vi "HFRR ADV v05 new software.vi"() -> ()   [LabVIEW 2025] (continued)
        n806 = local read "LIVE FEED MIN TEMP"() -> (w1181:bool)
        n807 = local write "LIVE FEED MAX TEMP"(TRUE ("LIVE FEED MAX TEMP")) -> ()
        n808 = local read "CAMERA ROI MIN TEMP"() -> (w1179:bool)
        n809 = case shown="True" w1181 {
          selector: w1181 -> [_ w1188]
          frame False {
          }
          frame True {
            n810 = Not(x=w1188) -> (.not. x?=w1187:bool)
            n811 = local write "LIVE FEED MIN TEMP"(w1187) -> ()
            n812 = call "CAMERA LIVE FEED FGV.vi"("Enum - Menu"=CAMERA_LIVE_FEED_ENUM."CAMERA MINIMIZE") -> ()  [unwired: 9 in, 2 out]
          }
        }
        n813 = case shown="True" w1179 {
          selector: w1179 -> [_ w1185]
          frame False {
          }
          frame True {
            n814 = Not(x=w1185) -> (.not. x?=w1184:bool)
            n815 = local write "CAMERA ROI MIN TEMP"(w1184) -> ()
            n816 = call "IMAGE ANALYSIS.vi"("Enum"=POST_ANALYSIS_ENUM."MINIMIZE UI") -> ()  [unwired: 9 in, 2 out]
          }
        }
        n817 = local write "CAMERA ROI MAX TEMP"(TRUE ("CAMERA ROI MAX TEMP")) -> ()
      }
      frame "About" {
        n818 = local read "LIVE FEED MIN TEMP"() -> (w1191:bool)
        n819 = local write "LIVE FEED MAX TEMP"(TRUE ("LIVE FEED MAX TEMP")) -> ()
        n820 = local read "CAMERA ROI MIN TEMP"() -> (w1190:bool)
        n821 = case shown="True" w1191 {
          selector: w1191 -> [_ w1198]
          frame False {
          }
          frame True {
            n822 = Not(x=w1198) -> (.not. x?=w1197:bool)
            n823 = local write "LIVE FEED MIN TEMP"(w1197) -> ()
            n824 = call "CAMERA LIVE FEED FGV.vi"("Enum - Menu"=CAMERA_LIVE_FEED_ENUM."CAMERA MINIMIZE") -> ()  [unwired: 9 in, 2 out]
          }
        }
        n825 = case shown="True" w1190 {
          selector: w1190 -> [_ w1195]
          frame False {
          }
          frame True {
            n826 = Not(x=w1195) -> (.not. x?=w1194:bool)
            n827 = local write "CAMERA ROI MIN TEMP"(w1194) -> ()
            n828 = call "IMAGE ANALYSIS.vi"("Enum"=POST_ANALYSIS_ENUM."MINIMIZE UI") -> ()  [unwired: 9 in, 2 out]
          }
        }
        n829 = local write "CAMERA ROI MAX TEMP"(TRUE ("CAMERA ROI MIN TEMP")) -> ()
      }
      frame "Advance" {
        n830 = local read "LIVE FEED MIN TEMP"() -> (w1201:bool)
        n831 = local write "LIVE FEED MAX TEMP"(TRUE ("LIVE FEED MAX TEMP")) -> ()
        n832 = local read "CAMERA ROI MIN TEMP"() -> (w1199:bool)
        n833 = case shown="True" w1201 {
          selector: w1201 -> [_ w1208]
          frame False {
          }
          frame True {
            n834 = Not(x=w1208) -> (.not. x?=w1207:bool)
            n835 = local write "LIVE FEED MIN TEMP"(w1207) -> ()
            n836 = call "CAMERA LIVE FEED FGV.vi"("Enum - Menu"=CAMERA_LIVE_FEED_ENUM."CAMERA MINIMIZE") -> ()  [unwired: 9 in, 2 out]
          }
        }
        n837 = local write "CAMERA ROI MAX TEMP"(TRUE ("CAMERA ROI MAX TEMP")) -> ()
        n838 = case shown="True" w1199 {
          selector: w1199 -> [_ w1205]
          frame False {
          }
          frame True {
            n839 = Not(x=w1205) -> (.not. x?=w1204:bool)
            n840 = local write "CAMERA ROI MIN TEMP"(w1204) -> ()
            n841 = call "IMAGE ANALYSIS.vi"("Enum"=POST_ANALYSIS_ENUM."MINIMIZE UI") -> ()  [unwired: 9 in, 2 out]
          }
        }
      }
      frame "Mooha" {
        n842 = local read "LIVE FEED MIN TEMP"() -> (w1211:bool)
        n843 = local write "LIVE FEED MAX TEMP"(TRUE ("LIVE FEED MAX TEMP")) -> ()
        n844 = local read "CAMERA ROI MIN TEMP"() -> (w1209:bool)
        n845 = case shown="True" w1211 {
          selector: w1211 -> [_ w1218]
          frame False {
          }
          frame True {
            n846 = Not(x=w1218) -> (.not. x?=w1217:bool)
            n847 = local write "LIVE FEED MIN TEMP"(w1217) -> ()
            n848 = call "CAMERA LIVE FEED FGV.vi"("Enum - Menu"=CAMERA_LIVE_FEED_ENUM."CAMERA MINIMIZE") -> ()  [unwired: 9 in, 2 out]
          }
        }
        n849 = local write "CAMERA ROI MAX TEMP"(TRUE ("CAMERA ROI MAX TEMP")) -> ()
        n850 = case shown="True" w1209 {
          selector: w1209 -> [_ w1215]
          frame False {
          }
          frame True {
            n851 = Not(x=w1215) -> (.not. x?=w1214:bool)
            n852 = local write "CAMERA ROI MIN TEMP"(w1214) -> ()
            n853 = call "IMAGE ANALYSIS.vi"("Enum"=POST_ANALYSIS_ENUM."MINIMIZE UI") -> ()  [unwired: 9 in, 2 out]
          }
        }
      }
    }
    n854 = local read "Auto Start Test"() -> (w960:bool)
    n855 = case shown="True" "sign in temp" {
      frame False {
      }
      frame True {
        w997 = 1 ("y")
        n856 = local read "USERNAME"() -> (w1003:string)
        n857 = local read "USER ID"() -> (w1000:string)
        n858 = call <vilib>:"Trim Whitespace.vi"("string"=w1003) -> ("trimmed string"=w1002:string)  [unwired: 1 in]
        n859 = call <vilib>:"Trim Whitespace.vi"("string"=w1000) -> ("trimmed string"=w1001:string)  [unwired: 1 in]
        n860 = String Length(string=w1002) -> (length=w999:i32)
        n861 = String Length(string=w1001) -> (length=w998:i32)
        n862 = Greater?(x=w999, y=w997) -> (0:w996:bool)
        n863 = Greater?(x=w998, y=w997) -> (0:w995:bool)
        n864 = And(x=w996, y=w995) -> (x .and. y?=w994:bool)
        n865 = case shown="True" w994 {
          frame False {
            n866 = property on="Sign In" class="Bool (strict)"("DisabledEnum"=T13."Disabled" ("Disabled")) -> ()  [unwired: 2 in, 2 out]
          }
          frame True {
            n867 = property on="Sign In" class="Bool (strict)"("DisabledEnum"=T13."Enabled" ("Disabled")) -> ()  [unwired: 2 in, 2 out]
          }
        }
      }
    }
    n868 = local read "Air Temperature"() -> (w977:bool)
    n869 = local read "Coefficient Of Friction"() -> (w978:bool)
    n870 = case shown="False" w960 {
      frame False {
        n871 = local read "Auto stop temp"() -> (w991:bool)
        n872 = case shown="True" w991 {
          frame False {
          }
          frame True {
            n873 = local write "Auto Start Temp"(FALSE ("Auto Start Temp")) -> ()
          }
        }
      }
      frame True {
        "Auto stop temp" <- TRUE ("Auto stop temp")
      }
    }
    n874 = local read "Humidity"() -> (w976:bool)
    n875 = case shown="\"HOME\"" w988 {
      frame "HOME" {
        n876 = local write "main tab sub"(enum32{"Page 1", "Page 2"}."Page 1" ("main tab sub")) -> ()
      }
      frame Default {
        n877 = local write "main tab sub"(enum32{"Page 1", "Page 2"}."Page 2" ("main tab sub")) -> ()
      }
    }
    n878 = case shown="True" w987 {
      selector: w987 -> [_ w1323]
      frame False {
      }
      frame True {
        n879 = Not(x=w1323) -> (.not. x?=w1322:bool)
        n880 = local write "Sign In"(w1322) -> ()
        n881 = local write "Main Dashboard Buttons"(T1."Test Setup" ("Main Dashboard Buttons")) -> ()
      }
    }
    n882 = case shown="\"Numeric Display\", Default" "Num/Graph" {
      frame "Numeric Display", Default {
        n883 = property on="Single/Multiple" class="RadioBtnsControl (strict)"("Visible"=FALSE) -> ()  [unwired: 2 in, 2 out]
        n884 = property on="Single - Graph" class="Ring (strict)"("Visible"=FALSE) -> ()  [unwired: 2 in, 2 out]
        n885 = local write "Main Tab Display"(T4."Dashboard 1" ("Main Tab Display")) -> ()
      }
      frame "Graph Display" {
        n886 = property on="Single/Multiple" class="RadioBtnsControl (strict)"("Visible"=TRUE) -> ()  [unwired: 2 in, 2 out]
        n887 = case shown="\"Multiple\"" "Single/Multiple" {
          frame "Single ", Default {
            n888 = property on="Single - Graph" class="Ring (strict)"("Visible"=TRUE) -> ()  [unwired: 2 in, 2 out]
            n889 = local write "Main Tab Display"(T4."Dashboard 3" ("Main Tab Display")) -> ()
          }
          frame "Multiple" {
            n890 = property on="Single - Graph" class="Ring (strict)"("Visible"=FALSE) -> ()  [unwired: 2 in, 2 out]
            n891 = local write "Main Tab Display"(T4."Dashboard 2" ("Main Tab Display")) -> ()
          }
        }
      }
    }
    n892 = local read "Stroke"() -> (w975:bool)
    n893 = local read "USERNAME"() -> (w981:string)
    n894 = local read "USER ID"() -> (w980:string)
    n895 = case shown="True" w978 {
      selector: w978 -> [_ w1258]
      frame False {
      }
      frame True {
        n896 = Not(x=w1258) -> (.not. x?=w1257:bool)
        n897 = local write "Coefficient Of Friction"(w1257) -> ()
        n898 = local write "Tab Control 2"(T6."Coefficient Of Friction" ("Tab Control 2")) -> ()
      }
    }
    n899 = case shown="True" w977 {
      selector: w977 -> [_ w1255]
      frame False {
      }
      frame True {
        n900 = Not(x=w1255) -> (.not. x?=w1253:bool)
        n901 = local write "Air Temperature"(w1253) -> ()
        n902 = local write "Tab Control 2"(T6."Air Temperature" ("Tab Control 2")) -> ()
      }
    }
    n903 = local write "Operator ID"(w980) -> ()
    n904 = case shown="True" w975 {
      selector: w975 -> [_ w1249]
      frame False {
      }
      frame True {
        n905 = Not(x=w1249) -> (.not. x?=w1247:bool)
        n906 = local write "Stroke"(w1247) -> ()
        n907 = local write "Tab Control 2"(T6."Stroke" ("Tab Control 2")) -> ()
      }
    }
    n908 = local write "tested by"(w981) -> ()
    n909 = case shown="True" w976 {
      selector: w976 -> [_ w1252]
      frame False {
      }
      frame True {
        n910 = Not(x=w1252) -> (.not. x?=w1250:bool)
        n911 = local write "Humidity"(w1250) -> ()
        n912 = local write "Tab Control 2"(T6."Humidity" ("Tab Control 2")) -> ()
      }
    }
    n913 = case shown="\"Advance\"" "Main Dashboard Buttons" {
      tunnel: [T2."HOME" ("Main Tab") T2."Test Setup" ("Main Tab") T2."Acquire" ("Main Tab") T2."Adv Scar" ("Main Tab") T2."Adv Scar Report" ("Main Tab") T2."Compare Files" ("Main Tab") T2."About" ("Main Tab") T2."Advance" ("Main Tab")] -> w985
      frame "Home", Default {
      }
      frame "Test Setup" {
      }
      frame "Dashboard" {
      }
      frame "Imaging" {
      }
      frame "Report" {
      }
      frame "Analysis" {
      }
      frame "About" {
      }
      frame "Advance" {
      }
    }
    n914 = Wait (ms)(milliseconds to wait=u32 100) -> ()  [unwired: 1 out]
    n915 = local read "Main Tab Display"() -> (w979:T4)
    n916 = local write "Main Tab"(w985) -> ()
    n917 = case shown="\"Dashboard 3\"" w979 {
      frame "Dashboard 1", Default {
        n918 = property on="Reset Graph" class="Bool (strict)"("Visible"=FALSE) -> ()  [unwired: 2 in, 2 out]
      }
      frame "Dashboard 2" {
        n919 = property on="Reset Graph" class="Bool (strict)"("Visible"=TRUE) -> ()  [unwired: 2 in, 2 out]
      }
      frame "Dashboard 3" {
        n920 = property on="Reset Graph" class="Bool (strict)"("Visible"=TRUE) -> ()  [unwired: 2 in, 2 out]
      }
    }
    n921 = local read "SCAR MEASURMENT"() -> (w967:enum32{"Auto Scar", "Manual Scar"})
    n922 = local read "Humidity"() -> (w982:bool)
    n923 = local read "Cap Live Image"() -> (w964:bool)
    n924 = local read "Sample Temperature"() -> (w974:bool)
    n925 = local read "Air Temp vs Humidity"() -> (w972:bool)
    n926 = local read "Frequency"() -> (w973:bool)
    n927 = case shown="False" w982 {
      frame False {
        n928 = local write "Humidity On Command"(TRUE ("Humidity On Command")) -> ()
        n929 = case shown="True" "Humidity Off Command" {
          selector: "Humidity Off Command" -> [_ w1265]
          frame False {
          }
          frame True {
            n930 = stacked-sequence {
              frame #0 {
                n931 = local read "WriteHumidity"() -> (w1267:string[])
                n932 = Insert Into Array(array=w1267, new element="R;1" ("new element/subarray")) -> (w1268:string[])  [unwired: 1 in]
                n933 = local write "WriteHumidity"(w1268) -> ()
              }
              frame #1 {
                n934 = Wait (ms)(milliseconds to wait=u32 2000) -> ()  [unwired: 1 out]
              }
              frame #2 {
                n935 = local read "EVENT LOG"() -> (w1274:string)
                n936 = local read "WriteHumidity"() -> (w1271:string[])
                n937 = call "Event Log.vi"("Content"="Humidity Control Off" ("string"), "EVENT LOG"=w1274) -> ("EVENT LOG"=w1275:string)  [unwired: 8 in, 1 out]
                n938 = local write "EVENT LOG"(w1275) -> ()
                n939 = Insert Into Array(array=w1271, new element="R;1" ("new element/subarray")) -> (w1272:string[])  [unwired: 1 in]
                n940 = local write "WriteHumidity"(w1272) -> ()
              }
            }
            n941 = Not(x=w1265) -> (.not. x?=w1264:bool)
            n942 = local write "Humidity Off Command"(w1264) -> ()
          }
        }
      }
      frame True {
        n943 = local write "Humidity Off Command"(TRUE ("Humidity Off Command")) -> ()
        n944 = case shown="False" "Humidity On Command" {
          selector: "Humidity On Command" -> [_ w1279]
          frame False {
          }
          frame True {
            n945 = stacked-sequence {
              frame #0 {
                n946 = local read "Set Rh"() -> (w1285:dbl)
                n947 = Number To Fractional String(number=w1285, precision (6)=i16 2) -> (F-format string=w1286:string)  [unwired: 2 in]
                n948 = local read "WriteHumidity"() -> (w1283:string[])
                n949 = Concatenate Strings("M;" ("new element/subarray"), w1286) -> (w1284:string)
                n950 = Insert Into Array(array=w1283, new element=w1284) -> (w1282:string[])  [unwired: 1 in]
                n951 = local write "WriteHumidity"(w1282) -> ()
              }
              frame #1 {
                n952 = Wait (ms)(milliseconds to wait=u32 1500) -> ()  [unwired: 1 out]
              }
              frame #2 {
                (unwired) "% RH" ("string")
                (unwired) i16 2 ("precision (6)")
                (unwired) "M;" ("new element/subarray")
                n953 = local read "Set Rh"() -> (w1293:dbl)
                n954 = Number To Fractional String(number=w1293, precision (6)=i16 2) -> (F-format string=w1290:string)  [unwired: 2 in]
                n955 = local read "WriteHumidity"() -> (w1295:string[])
                n956 = Concatenate Strings("M;" ("new element/subarray"), w1290) -> (w1294:string)
                n957 = Concatenate Strings("Humidity Set to : " ("string"), w1290, "% RH" ("string")) -> (w1288:string)
                n958 = Insert Into Array(array=w1295, new element=w1294) -> (w1296:string[])  [unwired: 1 in]
                n959 = disable-structure shown="Enabled" {
                  frame Enabled {
                    n960 = local read "EVENT LOG"() -> (w1299:string)
                    n961 = call "Event Log.vi"("Content"="Humidity Control On", "EVENT LOG"=w1299) -> ("EVENT LOG"=w1300:string)  [unwired: 8 in, 1 out]
                    n962 = local write "EVENT LOG"(w1300) -> ()
                  }
                  frame Disabled {
                  }
                }
                n963 = disable-structure shown="Enabled" {
                  disable-tunnel: w1288 -> [_ _]
                  frame Enabled {
                    n964 = local read "EVENT LOG"() -> (w1302:string)
                    n965 = call "Event Log.vi"("Content"="Humidity Control On", "EVENT LOG"=w1302) -> ("EVENT LOG"=w1303:string)  [unwired: 8 in, 1 out]
                    n966 = local write "EVENT LOG"(w1303) -> ()
                  }
                  frame Disabled {
                  }
                }
                n967 = local write "WriteHumidity"(w1296) -> ()
              }
            }
            n968 = Not(x=w1279) -> (.not. x?=w1278:bool)
            n969 = local write "Humidity On Command"(w1278) -> ()
          }
        }
      }
    }
    n970 = Equal?(x=w967, y=enum32{"Auto Scar", "Manual Scar"}."Auto Scar" ("SCAR MEASURMENT")) -> (x = y?=w963:bool)
    n971 = local read "TEST STANDARD"() -> (w970:T3)
    n972 = And(x=w964, y=w963) -> (x .and. y?=w965:bool)
    n973 = case shown="True" w965 {
      selector: w965 -> [_ w1064]
      tunnel: errorcluster {"status"=FALSE, "code"=0, "source"=""} ("error in (no error) 3") -> [_ w1065]
      frame False {
      }
      frame True {
        n974 = stacked-sequence {
          tunnel: w1065 -> [_ _ _ _ _ _ _ w1113]
          tunnel: w1064 -> [_ _ _ _ _ w1094 _ _]
          frame #0 {
            n975 = call "CAMERA LIVE FEED FGV.vi"("Enum - Menu"=CAMERA_LIVE_FEED_ENUM."CAMERA MINIMIZE") -> ()  [unwired: 9 in, 2 out]
          }
          frame #1 {
            n976 = property on="Auto Scar Check  2" class="Clust (strict)"("Visible"=TRUE) -> ()  [unwired: 2 in, 2 out]
          }
          frame #2 {
            n977 = String To Path(string="C:\\LAB-IQ\\Image Calibrate v01.dcf") -> (path=w1070:path)
            n978 = Open/Create/Replace File ("Open File")(file path (use dialog)=w1070) -> (refnum out=w1071:refnum<file>)  [unwired: 5 in, 2 out]
            n979 = for {
              N: 4 -> [_]
              tunnel: w1071 -> [w1077]
              i -> [w1073]
              n980 = Read from Text File ("Read File")(file (use dialog)=w1077) -> (text=w1078:string)  [unwired: 3 in, 3 out]
              n981 = String Subset(string=w1078, offset (0)=6, length (rest)=10 ("length (rest)")) -> (substring=w1074:string)
              n982 = Fract/Exp String To Number(string=w1074) -> (number=w1072:dbl)  [unwired: 3 in, 1 out]
              n983 = case shown="0" w1073 {
                tunnel: w1072 -> [w1079 w1080 _ w1081 _]
                frame 0 {
                  "5x Gain" <- w1079
                }
                frame 1 {
                  "10x Gain" <- w1080
                }
                frame 2 {
                }
                frame 3 {
                  "100x gain" <- w1081
                }
                frame 4, Default {
                }
              }
            }
          }
          frame #3 {
            n984 = local read "FILE 3"() -> (w1087:string)
            n985 = call <vilib>:"Trim Whitespace.vi"("string"="C:\\LAB-IQ\\images\\") -> ("trimmed string"=w1089:string)  [unwired: 1 in]
            n986 = String To Path(string=w1089) -> (path=w1088:path)
            n987 = Concatenate Strings(w1087, ".png" ("string")) -> (w1086:string)
            n988 = Build Path(base path=w1088, name or relative path=w1086) -> (appended path=w1084:path)
            "Image path" <- w1084
            n989 = Path To String(path=w1084) -> (string=w1083:string)
            n990 = call "CAMERA LIVE FEED FGV.vi"("Enum - Menu"=CAMERA_LIVE_FEED_ENUM."CAMERA SAVE", "Image Path"=w1083) -> ()  [unwired: 8 in, 2 out]
          }
          frame #4 {
            n991 = One Button Dialog(message="Image saved successfully") -> ()  [unwired: 1 in, 1 out]
          }
          frame #5 {
            n992 = local read "TEST STANDARD"() -> (w1093:T3)
            n993 = local read "Magnification len live scar"() -> (w1105:string)
            n994 = Not(x=w1094) -> (.not. x?=w1095:bool)
            n995 = local write "Cap Live Image"(w1095) -> ()
            n996 = case shown="\"ISO 12156\"" w1093 {
              tunnel: ["ASTM D6079" "ISO 12156"] -> w1092
              frame "ASTM D6079", Default {
              }
              frame "ISO 12156" {
              }
            }
            n997 = case shown="\"5x\", Default" w1105 {
              tunnel: [w1108 w1109] -> w1104
              frame "5x", Default {
                n998 = local read "5x Gain"() -> (w1108:dbl)
              }
              frame "10x" {
                # "5x"
                n999 = local read "10x Gain"() -> (w1109:dbl)
              }
            }
            n1000 = local read "Image path"() -> (w1103:path)
            n1001 = local read "FILE 3"() -> (w1096:string)
            n1002 = call "EDGE DETCTION.vi"("GAIN VALUE"=w1104, "Image Path"=w1103) -> ("error out"=w1102:errorcluster, "return value"=w1101:cluster{string, string, dbl, dbl, dbl})  [unwired: 8 in]
            n1003 = Bundle By Name(cluster=T18 {"File Name"="", "Test Method"="", "Operator"="", "Fuel Description"="", "Date and time"=""} ("Main Ref"), "File Name"=w1096, "Test Method"=w1092) -> (w1097:T18)
            n1004 = call "duf file read.vi"("error in (no error)"=w1102, "Main Ref"=w1097) -> ("error out"=w1100:errorcluster, "Main Ref 2"=w1098:T18)  [unwired: 8 in]
            n1005 = call "EDGE DETECTION REPORT.vi"("error in (no error)"=w1100, "return value 2"=w1101, "Main Ref"=w1098) -> ()  [unwired: 8 in, 1 out]
          }
          frame #6 {
            n1006 = property on="Auto Scar Check  2" class="Clust (strict)"("Visible"=FALSE) -> ()  [unwired: 2 in, 2 out]
          }
          frame #7 {
            n1007 = call "CAMERA LIVE FEED FGV.vi"("Enum - Menu"=CAMERA_LIVE_FEED_ENUM."CAMERA MINIMIZE", "error in (no error)"=w1113) -> ()  [unwired: 8 in, 2 out]
            n1008 = local write "Main Dashboard Buttons"(T1."Home" ("Main Dashboard Buttons")) -> ()
            n1009 = local write "Main Tab"(T2."HOME" ("Main Tab")) -> ()
          }
        }
      }
    }
    n1010 = local read "Heater Button"() -> (w971:bool)
    n1011 = case shown="True" w973 {
      selector: w973 -> [_ w1243]
      frame False {
      }
      frame True {
        n1012 = Not(x=w1243) -> (.not. x?=w1241:bool)
        n1013 = local write "Frequency"(w1241) -> ()
        n1014 = local write "Tab Control 2"(T6."Frequency" ("Tab Control 2")) -> ()
      }
    }
    n1015 = case shown="True" w972 {
      selector: w972 -> [_ w1240]
      frame False {
      }
      frame True {
        n1016 = Not(x=w1240) -> (.not. x?=w1238:bool)
        n1017 = local write "Air Temp vs Humidity"(w1238) -> ()
        n1018 = local write "Tab Control 2"(T6."Air Temp vs Rh" ("Tab Control 2")) -> ()
      }
    }
    n1019 = case shown="True" w974 {
      selector: w974 -> [_ w1246]
      frame False {
      }
      frame True {
        n1020 = Not(x=w1246) -> (.not. x?=w1244:bool)
        n1021 = local write "Sample Temperature"(w1244) -> ()
        n1022 = local write "Tab Control 2"(T6."Sample Temperature" ("Tab Control 2")) -> ()
      }
    }
    n1023 = case shown="\"Custom\"" w970 {
      frame "ASTM D6079", Default {
        w1219 = "ASTM D6079 TEST CONDITIONS" ("Standard 2")
        n1024 = local write "Standard 2"(w1219) -> ()
        n1025 = local write "Standard"(w1219) -> ()
      }
      frame "ISO 12156" {
        w1220 = "ISO 12156 TEST CONDITIONS" ("Standard 2")
        n1026 = local write "Standard 2"(w1220) -> ()
        n1027 = local write "Standard"(w1220) -> ()
      }
      frame "CEC F-096-A-06" {
        w1221 = "CEC F-096-A-06 TEST CONDITIONS" ("Standard 2")
        n1028 = local write "Standard 2"(w1221) -> ()
        n1029 = local write "Standard"(w1221) -> ()
      }
      frame "Custom" {
        w1222 = "CUSTOM TEST CONDITIONS" ("Standard 2")
        n1030 = local write "Standard 2"(w1222) -> ()
        n1031 = local write "Standard"(w1222) -> ()
      }
    }
    n1032 = case shown="True" w971 {
      frame False {
        n1033 = local write "Temperature On Command"(TRUE ("Temperature On Command")) -> ()
        n1034 = case shown="True" "Temperature Off Command" {
          selector: "Temperature Off Command" -> [_ w1226]
          frame False {
          }
          frame True {
            n1035 = Not(x=w1226) -> (.not. x?=w1225:bool)
            n1036 = local read "EVENT LOG"() -> (w1229:string)
            n1037 = local write "Temperature Off Command"(w1225) -> ()
            n1038 = call "Event Log.vi"("Content"="Heater Off", "EVENT LOG"=w1229) -> ("EVENT LOG"=w1228:string)  [unwired: 8 in, 1 out]
            n1039 = local write "EVENT LOG"(w1228) -> ()
          }
        }
      }
      frame True {
        n1040 = local write "Temperature Off Command"(TRUE ("Temperature Off Command")) -> ()
        n1041 = case shown="True" "Temperature On Command" {
          selector: "Temperature On Command" -> [_ w1233]
          frame False {
          }
          frame True {
            n1042 = Not(x=w1233) -> (.not. x?=w1232:bool)
            n1043 = local write "Temperature On Command"(w1232) -> ()
            n1044 = disable-structure shown="Enabled" {
              disable-tunnel: "Heater On" -> [w1235 _]
              frame Enabled {
                n1045 = local read "EVENT LOG"() -> (w1236:string)
                n1046 = call "Event Log.vi"("Content"=w1235, "EVENT LOG"=w1236) -> ("EVENT LOG"=w1237:string)  [unwired: 8 in, 1 out]
                n1047 = local write "EVENT LOG"(w1237) -> ()
              }
              frame Disabled {
              }
            }
          }
        }
      }
    }
    n1048 = local read "Main Tab"() -> (w962:T2)
    n1049 = case shown="\"About\"" w962 {
      frame "HOME", Default {
        w1008 = T13."Enabled" ("Disabled")
        n1050 = local read "Service Password enable"() -> (w1007:bool)
        n1051 = property on="Imaging" class="Bool (strict)"("DisabledEnum"=w1008) -> ()  [unwired: 2 in, 2 out]
        n1052 = property on="Dashboard" class="Bool (strict)"("DisabledEnum"=w1008) -> ()  [unwired: 2 in, 2 out]
        n1053 = property on="Test Setup" class="Bool (strict)"("DisabledEnum"=w1008) -> ()  [unwired: 2 in, 2 out]
        n1054 = property on="Analysis" class="Bool (strict)"("DisabledEnum"=w1008) -> ()  [unwired: 2 in, 2 out]
        n1055 = property on="Home" class="Bool (strict)"("DisabledEnum"=w1008) -> ()  [unwired: 2 in, 2 out]
        n1056 = property on="Report" class="Bool (strict)"("DisabledEnum"=w1008) -> ()  [unwired: 2 in, 2 out]
        n1057 = property on="Main Dashboard Buttons" class="RadioBtnsControl (strict)"("DisabledEnum"=w1008) -> ()  [unwired: 2 in, 2 out]
        n1058 = case shown="True" w1007 {
          tunnel: [T13."Disabled" ("Disabled") T13."Enabled" ("Disabled")] -> w1006
          frame False {
          }
          frame True {
          }
        }
        n1059 = property on="About" class="Bool (strict)"("DisabledEnum"=w1006) -> ()  [unwired: 2 in, 2 out]
      }
      frame "Test Setup" {
        w1013 = T13."Enabled" ("Disabled")
        n1060 = local read "Service Password enable"() -> (w1012:bool)
        n1061 = property on="Dashboard" class="Bool (strict)"("DisabledEnum"=T13."Disabled" ("Disabled")) -> ()  [unwired: 2 in, 2 out]
        n1062 = property on="Imaging" class="Bool (strict)"("DisabledEnum"=w1013) -> ()  [unwired: 2 in, 2 out]
        n1063 = property on="Analysis" class="Bool (strict)"("DisabledEnum"=w1013) -> ()  [unwired: 2 in, 2 out]
        n1064 = property on="Home" class="Bool (strict)"("DisabledEnum"=w1013) -> ()  [unwired: 2 in, 2 out]
        n1065 = property on="Report" class="Bool (strict)"("DisabledEnum"=w1013) -> ()  [unwired: 2 in, 2 out]
        n1066 = property on="Test Setup" class="Bool (strict)"("DisabledEnum"=w1013) -> ()  [unwired: 2 in, 2 out]
        n1067 = case shown="True" w1012 {
          tunnel: [T13."Disabled" ("Disabled") T13."Enabled" ("Disabled")] -> w1011
          frame False {
          }
          frame True {
          }
        }
        n1068 = property on="About" class="Bool (strict)"("DisabledEnum"=w1011) -> ()  [unwired: 2 in, 2 out]
      }
      frame "Adv Scar" {
        w1020 = T13."Enabled" ("Disabled")
        n1069 = property on="Dashboard" class="Bool (strict)"("DisabledEnum"=T13."Disabled" ("Disabled")) -> ()  [unwired: 2 in, 2 out]
        n1070 = property on="Imaging" class="Bool (strict)"("DisabledEnum"=w1020) -> ()  [unwired: 2 in, 2 out]
        n1071 = property on="Analysis" class="Bool (strict)"("DisabledEnum"=w1020) -> ()  [unwired: 2 in, 2 out]
        n1072 = property on="Home" class="Bool (strict)"("DisabledEnum"=w1020) -> ()  [unwired: 2 in, 2 out]
        n1073 = property on="Report" class="Bool (strict)"("DisabledEnum"=w1020) -> ()  [unwired: 2 in, 2 out]
        n1074 = property on="Test Setup" class="Bool (strict)"("DisabledEnum"=w1020) -> ()  [unwired: 2 in, 2 out]
        n1075 = local read "Service Password enable"() -> (w1018:bool)
        n1076 = case shown="True" w1018 {
          tunnel: [T13."Disabled" ("Disabled") T13."Enabled" ("Disabled")] -> w1017
          frame False {
          }
          frame True {
          }
        }
        n1077 = property on="About" class="Bool (strict)"("DisabledEnum"=w1017) -> ()  [unwired: 2 in, 2 out]
      }
      frame "Adv Scar Report" {
        w1025 = T13."Enabled" ("Disabled")
        n1078 = property on="Dashboard" class="Bool (strict)"("DisabledEnum"=T13."Disabled" ("Disabled")) -> ()  [unwired: 2 in, 2 out]
        n1079 = property on="Imaging" class="Bool (strict)"("DisabledEnum"=w1025) -> ()  [unwired: 2 in, 2 out]
        n1080 = property on="Analysis" class="Bool (strict)"("DisabledEnum"=w1025) -> ()  [unwired: 2 in, 2 out]
        n1081 = property on="Home" class="Bool (strict)"("DisabledEnum"=w1025) -> ()  [unwired: 2 in, 2 out]
        n1082 = property on="Report" class="Bool (strict)"("DisabledEnum"=w1025) -> ()  [unwired: 2 in, 2 out]
        n1083 = property on="Test Setup" class="Bool (strict)"("DisabledEnum"=w1025) -> ()  [unwired: 2 in, 2 out]
        n1084 = local read "Service Password enable"() -> (w1024:bool)
        n1085 = case shown="True" w1024 {
          tunnel: [T13."Disabled" ("Disabled") T13."Enabled" ("Disabled")] -> w1023
          frame False {
          }
          frame True {
          }
        }
        n1086 = property on="About" class="Bool (strict)"("DisabledEnum"=w1023) -> ()  [unwired: 2 in, 2 out]
      }
      frame "Compare Files" {
        w1031 = T13."Enabled" ("Disabled")
        n1087 = local read "Service Password enable"() -> (w1030:bool)
        n1088 = property on="Dashboard" class="Bool (strict)"("DisabledEnum"=T13."Disabled" ("Disabled")) -> ()  [unwired: 2 in, 2 out]
        n1089 = property on="Imaging" class="Bool (strict)"("DisabledEnum"=w1031) -> ()  [unwired: 2 in, 2 out]
        n1090 = property on="Analysis" class="Bool (strict)"("DisabledEnum"=w1031) -> ()  [unwired: 2 in, 2 out]
        n1091 = property on="Home" class="Bool (strict)"("DisabledEnum"=w1031) -> ()  [unwired: 2 in, 2 out]
        n1092 = property on="Report" class="Bool (strict)"("DisabledEnum"=w1031) -> ()  [unwired: 2 in, 2 out]
        n1093 = property on="Test Setup" class="Bool (strict)"("DisabledEnum"=w1031) -> ()  [unwired: 2 in, 2 out]
        n1094 = case shown="True" w1030 {
          tunnel: [T13."Disabled" ("Disabled") T13."Enabled" ("Disabled")] -> w1029
          frame False {
          }
          frame True {
          }
        }
        n1095 = property on="About" class="Bool (strict)"("DisabledEnum"=w1029) -> ()  [unwired: 2 in, 2 out]
      }
      frame "Acquire" {
        n1096 = local read "Service Password enable"() -> (w1035:bool)
        n1097 = property on="Test Setup" class="Bool (strict)"("DisabledEnum"=T13."Disabled" ("Disabled")) -> ()  [unwired: 2 in, 2 out]
        n1098 = local read "Auto Start Test"() -> (w1037:bool)
        n1099 = local read "RUN"() -> (w1039:bool)
        n1100 = case shown="True" w1035 {
          tunnel: [T13."Disabled" ("Disabled") T13."Enabled" ("Disabled")] -> w1036
          frame False {
          }
          frame True {
          }
        }
        n1101 = Or(x=w1039, y=w1037) -> (x .or. y?=w1038:bool)
        n1102 = case shown="True" w1038 {
          tunnel: [T13."Enabled" ("Disabled") T13."Disabled" ("Disabled")] -> w1041
          frame False {
          }
          frame True {
          }
        }
        n1103 = property on="About" class="Bool (strict)"("DisabledEnum"=w1036) -> ()  [unwired: 2 in, 2 out]
        n1104 = property on="Imaging" class="Bool (strict)"("DisabledEnum"=w1041) -> ()  [unwired: 2 in, 2 out]
        n1105 = property on="Dashboard" class="Bool (strict)"("DisabledEnum"=w1041) -> ()  [unwired: 2 in, 2 out]
        n1106 = property on="Analysis" class="Bool (strict)"("DisabledEnum"=w1041) -> ()  [unwired: 2 in, 2 out]
        n1107 = property on="Home" class="Bool (strict)"("DisabledEnum"=w1041) -> ()  [unwired: 2 in, 2 out]
        n1108 = property on="Report" class="Bool (strict)"("DisabledEnum"=w1041) -> ()  [unwired: 2 in, 2 out]
      }
      frame "About" {
        n1109 = local read "FILE"() -> (w1054:string)
        n1110 = local read "TEST FILE NAM,E SAVED"() -> (w1047:bool)
        n1111 = call <vilib>:"Trim Whitespace.vi"("string"=w1054) -> ("trimmed string"=w1053:string)  [unwired: 1 in]
        n1112 = local read "Auto Start Test"() -> (w1057:bool)
        n1113 = String Length(string=w1053) -> (length=w1052:i32)
        n1114 = Greater?(x=w1052, y=1) -> (0:w1049:bool)
        n1115 = And(x=w1049, y=w1047) -> (x .and. y?=w1048:bool)
        n1116 = local read "RUN"() -> (w1059:bool)
        n1117 = case shown="True" w1048 {
          tunnel: [T13."Disabled" ("Disabled") T13."Enabled" ("Disabled")] -> w1050
          frame False {
          }
          frame True {
          }
        }
        n1118 = Or(x=w1059, y=w1057) -> (x .or. y?=w1058:bool)
        n1119 = property on="About" class="Bool (strict)"("DisabledEnum"=T13."Enabled" ("Disabled")) -> ()  [unwired: 2 in, 2 out]
        n1120 = case shown="False" w1058 {
          tunnel: [T13."Enabled" ("Disabled") T13."Disabled" ("Disabled")] -> w1056
          frame False {
          }
          frame True {
          }
        }
        n1121 = property on="Dashboard" class="Bool (strict)"("DisabledEnum"=w1050) -> ()  [unwired: 2 in, 2 out]
        n1122 = property on="Test Setup" class="Bool (strict)"("DisabledEnum"=T13."Disabled" ("Disabled")) -> ()  [unwired: 2 in, 2 out]
        n1123 = property on="Imaging" class="Bool (strict)"("DisabledEnum"=w1056) -> ()  [unwired: 2 in, 2 out]
        n1124 = property on="Analysis" class="Bool (strict)"("DisabledEnum"=w1056) -> ()  [unwired: 2 in, 2 out]
        n1125 = property on="Home" class="Bool (strict)"("DisabledEnum"=w1056) -> ()  [unwired: 2 in, 2 out]
        n1126 = property on="Report" class="Bool (strict)"("DisabledEnum"=w1056) -> ()  [unwired: 2 in, 2 out]
      }
    }
    n1127 = local read "Quit"() -> (w990:bool)
    "Single" <- "Single - Graph"
  }
  n1128 = disable-structure shown="Disabled" {
    disable-tunnel: [w1327 _] -> w39
    disable-tunnel: _ -> [w1326 _]
    frame Disabled {
      n1129 = while {
        tunnel: w1326 -> [_]
        tunnel: [w1328] -> w1327
        tunnel: [w1329] -> _
        i -> [w1329]
        stop <- w1328 stop-if-true
        w1345 = u16 10 items=["1.0"=10, "1.5"=15, "2.0"=20] ("stop bits (10: 1 bit)")
        n1130 = Wait (ms)(milliseconds to wait=u32 10) -> ()  [unwired: 1 out]
        n1131 = call-poly "VISA Configure Serial Port"("VISA resource name"=refnum<visa-resource-name> "ASRL1::INSTR" ("COM PORT"), "timeout (10sec)"=u32 10, "baud rate (9600)"=u32 57600, "data bits (8)"=u16 8, "stop bits (10: 1 bit)"=w1345) -> ("VISA resource name out"=w1331:refnum<visa-resource-name>, "error out"=w1340:errorcluster)  [unwired: 9 in]
        n1132 = VISA Read(VISA resource name=w1331, byte count=u32 2 ("byte count (0)")) -> (read buffer=w1339:string)  [unwired: 1 in, 3 out]
        n1133 = String Subset(string=w1339, offset (0)=0, length (rest)=2 ("length (rest)")) -> (substring=w1338:string)
        n1134 = Match Pattern(string=w1338, regular expression="<>") -> (offset past match=w1335:i32)  [unwired: 1 in, 3 out]
        n1135 = Greater Or Equal?(x=w1335, y=0) -> (x >= y?=w1330:bool)
        n1136 = case shown="True" w1330 {
          tunnel: w1331 -> [_ w1349]
          tunnel: w1340 -> [_ w1348]
          frame False {
          }
          frame True {
            n1137 = VISA Read(VISA resource name=w1349, byte count=u32 32 ("byte count (0)"), error in (no error)=w1348) -> (read buffer=w1347:string)  [unwired: 3 out]
            n1138 = String Subset(string=w1347, offset (0)=0, length (rest)=8 ("length (rest)")) -> (substring=w1351:string)
            n1139 = String Subset(string=w1347, offset (0)=8, length (rest)=8 ("length (rest)")) -> (substring=w1352:string)
            n1140 = Decimal String To Number(string=w1352) -> (number=w1359:i32)  [unwired: 2 in, 1 out]
            n1141 = Decimal String To Number(string=w1351) -> (number=w1355:i32)  [unwired: 2 in, 1 out]
            n1142 = Divide(x=w1359, y=10000) -> ()  [unwired: 1 out]
            n1143 = Divide(x=w1355, y=1000000) -> ()  [unwired: 1 out]
          }
        }
        n1144 = local read "Quit"() -> (w1328:bool)
      }
    }
    frame Enabled {
    }
  }
  n1145 = while {
    shift-right: [w1374] -> w52
    shift-left: _ -> [w1365]
    shift-right: [w1373] -> w51
    shift-left: errorcluster {"status"=TRUE, "code"=0, "source"="Init"} ("error IO") -> [w1367]
    tunnel: [w1362] -> w42
    tunnel: [w1372] -> _
    i -> [w1372]
    stop <- w1362 stop-if-true
    n1146 = local read "Port 1a"() -> (w1368:bool)
    n1147 = local read "Port 3"() -> (w1369:bool)
    n1148 = local read "Com Port 1"() -> (w1366:refnum<visa-resource-name>)
    n1149 = Or(x=w1369, y=w1368) -> (x .or. y?=w1371:bool)
    n1150 = Unbundle(w1367) -> ("status"=→"Port 3":bool)  [unwired: 2 out]
    n1151 = Not Equal?(x=w1366, y=w1365) -> (x != y?=w1363:bool)
    n1152 = case shown="True" w1371 {
      frame False {
        w1377 = FALSE ("Visible")
        n1153 = property on="Port 1a" class="Bool (strict)"("Visible"=w1377) -> ()  [unwired: 2 in, 2 out]
        n1154 = property on="Port 3" class="Bool (strict)"("Visible"=w1377) -> ()  [unwired: 2 in, 2 out]
      }
      frame True {
        w1378 = TRUE ("Visible")
        n1155 = property on="Port 1a" class="Bool (strict)"("Visible"=w1378) -> ()  [unwired: 2 in, 2 out]
        n1156 = property on="Port 3" class="Bool (strict)"("Visible"=w1378) -> ()  [unwired: 2 in, 2 out]
      }
    }
    n1157 = Wait (ms)(milliseconds to wait=u32 40) -> ()  [unwired: 1 out]
    n1158 = case shown="True" w1363 {
      tunnel: [w1375 errorcluster {"status"=TRUE, "code"=0, "source"="Init"} ("error out")] -> w1364
      tunnel: w1367 -> [w1375 _]
      frame False {
      }
      frame True {
      }
    }
    n1159 = case shown="No Error" w1364 {
      selector: w1364 -> [w1386 w1413]
      tunnel: [w1379 w1417] -> w1374
      tunnel: [w1388 w1411] -> w1373
      tunnel: w1365 -> [w1387 w1415]
      frame No Error {
        n1160 = property class="Instr"(reference=w1387, error in=w1386) -> (reference out=w1384:refnum<visa-resource-name>, error out=w1385:errorcluster, "Serial Settings:Number of Bytes at Serial Port"=w1380:u32)
        n1161 = Greater?(x=w1380, y=u32 5) -> (0:w1382:bool)
        n1162 = Not(x=w1382) -> (.not. x?=→"Port 1a":bool)
        n1163 = while {
          tunnel: [w1406] -> w1388
          tunnel: [w1405] -> w1389
          tunnel: w1385 -> [w1404]
          tunnel: w1384 -> [w1403]
          stop <- TRUE stop-if-true
          n1164 = property class="Instr" props=["Serial Settings:Number of Bytes at Serial Port"](reference=w1403, error in=w1404) -> (reference out=w1408:refnum<visa-resource-name>, error out=w1407:errorcluster)  [unwired: 1 out]
          n1165 = VISA Read(VISA resource name=w1408, byte count=u32 50, error in (no error)=w1407) -> (VISA resource name out=w1405:refnum<visa-resource-name>, read buffer=w1390:string, error out=w1406:errorcluster)  [unwired: 1 out]
          "UNI READ" <- w1390
          n1166 = Spreadsheet String To Array(delimiter (Tab)=";", format string="", spreadsheet string=w1390, array type (2D Dbl)=dbl[] []) -> (array=w1400:dbl[])
          n1167 = Index Array(array=w1400) -> (element #1=→"LVDT MIN":dbl, element #2=→"LVDT MAX":dbl, element #3=→"LVDT Peak":dbl, element #4=→"pizo raw":dbl, element #5=→"Friction":dbl, element #6=→"cof 2":dbl)  [unwired: 6 in]
        }
        n1168 = VISA Flush I/O Buffer(VISA resource name=w1389) -> (VISA resource name out=w1379:refnum<visa-resource-name>)  [unwired: 2 in, 1 out]
      }
      frame Error {
        w1423 = u16 0 items=["None", "XON/XOFF", "RTS/CTS", "XON/XOFF & RTS/CTS", "DTR/DSR", "XON/XOFF & DTR/DSR"] ("flow control (0:none)  2")
        w1421 = u16 10 items=["1.0"=10, "1.5"=15, "2.0"=20] ("stop bits 2")
        w1419 = u16 0 items=["None", "Odd", "Even", "Mark", "Space"] ("parity 2")
        w1420 = u32 10000  # timeout (10sec)
        n1169 = VISA Close(VISA resource name=w1415, error in (no error)=w1413) -> (error out=w1416:errorcluster)
        n1170 = local write "Port 1a"(FALSE ("Port 1a")) -> ()
        n1171 = local read "Com Port 1"() -> (w1410:refnum<visa-resource-name>)
        n1172 = call <vilib>:"Clear Errors.vi"("error in (no error)"=w1416) -> ("error out"=w1414:errorcluster)  [unwired: 5 in, 1 out]
        n1173 = call-poly "VISA Configure Serial Port"("VISA resource name"=w1410, "timeout (10sec)"=w1420, "baud rate (9600)"=u32 250000 ("baud rate  2"), "data bits (8)"=u16 8 ("data bits  2"), "parity (0:none)"=w1419, "error in (no error)"=w1414, "stop bits (10: 1 bit)"=w1421, "flow control (0:none)"=w1423) -> ("VISA resource name out"=w1424:refnum<visa-resource-name>, "error out"=w1425:errorcluster)  [unwired: 6 in]
        n1174 = flat-sequence {
          tunnel: w1424 -> [w1427]
          tunnel: w1425 -> [w1426]
          tunnel: [w1427] -> w1417
          tunnel: [w1426] -> w1411
          frame #0 {
            n1175 = Wait (ms)(milliseconds to wait=u32 50) -> ()  [unwired: 1 out]
          }
        }
        "Residual Uno" <- ""
        "Port 1 Error" <- w1411
      }
    }
    n1176 = local read "Quit"() -> (w1362:bool)
    "Error Uno" <- w1367
  }
  n1177 = while {
    stop <- w1434 stop-if-true
    # "V0OLTAGE TO STROKE (peice vise calibration)"
    n1178 = Wait (ms)(milliseconds to wait=u32 10) -> ()  [unwired: 1 out]
    n1179 = local read "LVDT Peak"() -> (w1431:dbl)
    n1180 = formula code="// Dynamic Parameterized Linear Interpolation Node\n// Inputs: vpp_val, voltages (Array), distances (Array)\n// Outputs: stroke\n\nint i = 0;\nint segments = 11; // 12 points make 11 interpolation segments\n\n// 1. Lower Boundary Clamp\nif (vpp_val <= voltages[0]) {\n    stroke = distances[0];\n}\n// 2. Upper Boundary Clamp\nelse if (vpp_val >= voltages[segments]) {\n    stroke = distances[segments];\n}\n// 3. Dynamic Segment Search Loop\nelse {\n    stroke = distances[0]; // Fallback baseline\n    for (i = 0; i < segments; i++) {\n        if (vpp_val >= voltages[i] && vpp_val <= voltages[i+1]) {\n            // Standard linear interpolation formula using array lookups\n            stroke = distances[i] + (vpp_val - voltages[i]) * (distances[i+1] - distances[i]) / (voltages[i+1] - voltages[i]);\n            break; // Segment found, safely exit the loop\n        }\n    }\n}"("vpp_val"=w1431, "voltages"="calibration values", "distances"="STROKE") -> ("stroke"=→"LVDT STROKE":dbl)
    n1181 = local read "Quit"() -> (w1434:bool)
  }
  n1182 = while {
    stop <- w1454 stop-if-true
    n1183 = call <vilib>:"High Resolution Polling Wait.vi"("seconds to wait"=0.02) -> ()  [unwired: 10 in, 1 out]
    n1184 = local read "Due read"() -> (w1452:string)
    n1185 = Spreadsheet String To Array(delimiter (Tab)=";", format string="", spreadsheet string=w1452, array type (2D Dbl)=string[] []) -> (array=w1449:string[])
    n1186 = Fract/Exp String To Number(string=w1449) -> (number=w1448:dbl[])  [unwired: 3 in, 1 out]
    n1187 = Index Array(array=w1448) -> (element #1=→"Sample Temperature":dbl, element #2=→"Target Sample Temperature":dbl, element #3=→"Current Duty Cycle":dbl, element #4=→"Ambient Temperature":dbl, element #5=→"Dac Status":dbl, element #6=→"Vpp":dbl, element #7=→"Active Error Code":dbl, element #8=→"Kp":dbl, element #9=→"Ki":dbl, element #10=→"Kd":dbl, element #11=→"SampleRaw":dbl, element #12=→"AmbRaw":dbl)  [unwired: 12 in]
    n1188 = local read "Quit"() -> (w1454:bool)
  }
  n1189 = while {
    shift-right: [w1468] -> w37
    shift-left: _ -> [w1459]
    shift-right: [w1467] -> w36
    shift-left: errorcluster {"status"=FALSE, "code"=0, "source"="Init"} ("error out") -> [w1461]
    tunnel: [w1456] -> w41
    tunnel: [w1466] -> _
    i -> [w1466]
    stop <- w1456 stop-if-true
    n1190 = local read "Com Port 2"() -> (w1460:refnum<visa-resource-name>)
    n1191 = local read "Port 2a"() -> (w1462:bool)
    n1192 = Unbundle(w1461) -> ("status"=→"Port 4":bool)  [unwired: 2 out]
    n1193 = call <vilib>:"High Resolution Polling Wait.vi"("seconds to wait"=0.02) -> ()  [unwired: 10 in, 1 out]
    n1194 = local read "Port 4"() -> (w1463:bool)
    n1195 = Not Equal?(x=w1460, y=w1459) -> (x != y?=w1458:bool)
    n1196 = Or(x=w1463, y=w1462) -> (x .or. y?=w1465:bool)
    n1197 = case shown="True" w1465 {
      frame False {
        w1471 = FALSE ("Visible")
        n1198 = property on="Port 2a" class="Bool (strict)"("Visible"=w1471) -> ()  [unwired: 2 in, 2 out]
        n1199 = property on="Port 4" class="Bool (strict)"("Visible"=w1471) -> ()  [unwired: 2 in, 2 out]
      }
      frame True {
        w1472 = TRUE ("Visible")
        n1200 = property on="Port 2a" class="Bool (strict)"("Visible"=w1472) -> ()  [unwired: 2 in, 2 out]
        n1201 = property on="Port 4" class="Bool (strict)"("Visible"=w1472) -> ()  [unwired: 2 in, 2 out]
      }
    }
    n1202 = case shown="True" w1458 {
      tunnel: [w1469 errorcluster {"status"=TRUE, "code"=0, "source"="Init"} ("error out")] -> w1457
      tunnel: w1461 -> [w1469 _]
      frame False {
      }
      frame True {
      }
    }
    n1203 = case shown="No Error" w1457 {
      selector: w1457 -> [w1483 w1514]
      tunnel: [w1476 w1519] -> w1468
      tunnel: [w1484 w1512] -> w1467
      tunnel: w1459 -> [w1486 w1517]
      frame No Error {
        n1204 = property class="Instr" props=["Serial Settings:Number of Bytes at Serial Port"](reference=w1486, error in=w1483) -> (reference out=w1477:refnum<visa-resource-name>, error out=w1482:errorcluster)  [unwired: 1 out]
        n1205 = while {
          tunnel: [w1494] -> w1478
          tunnel: [w1493] -> w1479
          tunnel: w1482 -> [w1492]
          tunnel: w1477 -> [w1491]
          tunnel: [w1490] -> _
          i -> [w1490]
          stop <- TRUE stop-if-true
          n1206 = property class="Instr" props=["Serial Settings:Number of Bytes at Serial Port"](reference=w1491, error in=w1492) -> (reference out=w1496:refnum<visa-resource-name>, error out=w1495:errorcluster)  [unwired: 1 out]
          n1207 = VISA Read(VISA resource name=w1496, byte count=u32 1000, error in (no error)=w1495) -> (VISA resource name out=w1493:refnum<visa-resource-name>, read buffer=→"Due read":string, error out=w1494:errorcluster)  [unwired: 1 out]
        }
        n1208 = local read "Command"() -> (w1474:string)
        n1209 = call <vilib>:"Trim Whitespace.vi"("string"=w1474) -> ("trimmed string"=w1473:string)  [unwired: 1 in]
        n1210 = Not Equal?(x=w1473, y="") -> (x != y?=w1480:bool)
        n1211 = case shown="True" w1480 {
          tunnel: w1479 -> [w1498 w1503]
          tunnel: [w1498 w1507] -> w1485
          tunnel: w1478 -> [w1497 w1502]
          tunnel: [w1497 w1505] -> w1484
          tunnel: w1473 -> [_ w1501]
          tunnel: [_ w1504] -> _
          frame False {
            # "DATA  WRITE LOOP"
          }
          frame True {
            n1212 = Concatenate Strings(w1501, "\r\n") -> (w1500:string)
            n1213 = VISA Write(VISA resource name=w1503, write buffer=w1500, error in (no error)=w1502) -> (VISA resource name out=w1507:refnum<visa-resource-name>, return count=w1504:u32, error out=w1506:errorcluster)
            n1214 = flat-sequence {
              tunnel: w1506 -> [w1509]
              tunnel: [w1509] -> w1505
              frame #0 {
                n1215 = local write "Command"("" ("Command")) -> ()
                n1216 = Wait (ms)(milliseconds to wait=u32 5) -> ()  [unwired: 1 out]
              }
            }
          }
        }
        n1217 = VISA Flush I/O Buffer(VISA resource name=w1485) -> (VISA resource name out=w1476:refnum<visa-resource-name>, error out=→"error out 9":errorcluster)  [unwired: 2 in]
      }
      frame Error {
        w1525 = u16 0 items=["None", "XON/XOFF", "RTS/CTS", "XON/XOFF & RTS/CTS", "DTR/DSR", "XON/XOFF & DTR/DSR"] ("flow control (0:none)  2")
        w1523 = u16 10 items=["1.0"=10, "1.5"=15, "2.0"=20] ("stop bits 2")
        w1521 = u16 0 items=["None", "Odd", "Even", "Mark", "Space"] ("parity 2")
        w1522 = u32 10000  # timeout (10sec)
        n1218 = VISA Clear(VISA resource name=w1517, error in (no error)=w1514) -> (VISA resource name out=w1516:refnum<visa-resource-name>, error out=w1515:errorcluster)
        n1219 = VISA Close(VISA resource name=w1516, error in (no error)=w1515) -> (error out=w1518:errorcluster)
        n1220 = call <vilib>:"Clear Errors.vi"("error in (no error)"=w1518) -> ()  [unwired: 5 in, 2 out]
        n1221 = local read "Com Port 2"() -> (w1511:refnum<visa-resource-name>)
        "visa due" <- w1511
        n1222 = call-poly "VISA Configure Serial Port"("VISA resource name"=w1511, "timeout (10sec)"=w1522, "baud rate (9600)"=u32 250000 ("baud rate  2"), "data bits (8)"=u16 8 ("data bits  2"), "parity (0:none)"=w1521, "stop bits (10: 1 bit)"=w1523, "flow control (0:none)"=w1525) -> ("VISA resource name out"=w1526:refnum<visa-resource-name>, "error out"=w1527:errorcluster)  [unwired: 7 in]
        n1223 = flat-sequence {
          tunnel: w1526 -> [w1529]
          tunnel: w1527 -> [w1528]
          tunnel: [w1529] -> w1519
          tunnel: [w1528] -> w1512
          frame #0 {
            n1224 = Wait (ms)(milliseconds to wait=u32 50) -> ()  [unwired: 1 out]
          }
        }
        "Residual Due" <- ""
        "Port 2 Error" <- w1512
      }
    }
    n1225 = local read "Quit"() -> (w1456:bool)
    "Error Due" <- w1461
  }
  n1226 = local write "FRICVALZ"(0.0 ("FRICVALZ")) -> ()
  n1227 = property on="RUN" class="Bool (strict)"("Visible"=TRUE) -> ()  [unwired: 2 in, 2 out]
  n1228 = while {
    tunnel: [w1546] -> _
    tunnel: [w1531] -> w54
    i -> [w1546]
    stop <- w1531 stop-if-true
    n1229 = local read "conststatus"() -> (w1535:dbl)
    n1230 = local read "Main Tab"() -> (w1533:T2)
    n1231 = local read "EDIT"() -> (w1552:bool)
    n1232 = local read "Rate"() -> (w1551:dbl)
    n1233 = case shown="True" w1552 {
      tunnel: [FALSE TRUE] -> w1538
      frame False {
      }
      frame True {
      }
    }
    n1234 = property on="Time slide" class="Slide (strict)"("Scale.Range:Maximum"=2500.0) -> ()  [unwired: 2 in, 2 out]
    n1235 = Equal?(x=w1533, y=T20."About" ("Main Tab")) -> (x = y?=w1544:bool)
    n1236 = Equal?(x=w1535, y=0.0) -> (x = y?=w1536:bool)
    n1237 = Divide(x=1.0, y=w1551) -> (x/y=w1547:dbl)
    "Time 2" <- w1547
    n1238 = case shown="True" w1536 {
      frame False {
      }
      frame True {
        # "C:\\WinDucom\\calibrate WO 2391.dcf"
        n1239 = local write "Lan flag"(22) -> ()
        n1240 = local write "conststatus"(10.0 ("rpm value : 2")) -> ()
        n1241 = String To Path(string="C:\\LAB-IQ\\calibrate WO 2465.dcf") -> (path=w1558:path)
        n1242 = Open/Create/Replace File "Open File"(file path (use dialog)=w1558) -> (refnum out=w1556:refnum<file>)  [unwired: 5 in, 2 out]
        n1243 = for {
          N: 23 -> [_]
          tunnel: w1556 -> [w1567]
          i -> [w1561]
          (unwired) TRUE ("line mode (F)")
          n1244 = Read from Text File "Read File"(file (use dialog)=w1567) -> (text=w1566:string)  [unwired: 3 in, 3 out]
          n1245 = Match Pattern(string=w1566, regular expression="]") -> (after substring=w1564:string)  [unwired: 1 in, 3 out]
          n1246 = String Subset(string=w1566, offset (0)=5, length (rest)=10 ("length (rest)")) -> (substring=w1559:string)
          n1247 = Fract/Exp String To Number(string=w1559) -> (number=w1560:dbl)  [unwired: 3 in, 1 out]
          n1248 = Match Pattern(string=w1564, regular expression="-") -> (before substring=w1562:string)  [unwired: 1 in, 3 out]
          n1249 = case shown="4" w1561 {
            tunnel: w1560 -> [w1570 w1571 w1572 w1573 _ _ _ w1578 w1579 _ w1580 w1581 w1582 w1583 w1584 w1585 _ w1586 w1587 _ _ _ _ _]
            tunnel: w1562 -> [_ _ _ _ w1574 w1575 w1576 _ _ _ _ _ _ _ _ _ _ _ _ w1588 w1589 _ w1590 _]
            frame 0 {
              n1250 = local write "FRIC. FORCE :"(w1570) -> ()
            }
            frame 1 {
              n1251 = local write "TEMPERATURE :"(w1571) -> ()
            }
            frame 2 {
              n1252 = local write "HUMIDITY:"(w1572) -> ()
            }
            frame 3 {
              n1253 = local write "AIR TEMPERATURE :"(w1573) -> ()
            }
            frame 4 {
              n1254 = local write "Com Port 1"(w1574) -> ()
            }
            frame 5 {
              n1255 = local write "Com Port 2"(w1575) -> ()
              n1256 = local write "visa due"(w1575) -> ()
            }
            frame 6 {
              n1257 = String To Path(string=w1576) -> (path=w1577:path)
              n1258 = local write "File Path"(w1577) -> ()
              "String" <- w1576
            }
            frame 7 {
              n1259 = local write "DISPLACEMENT :"(w1578) -> ()
            }
            frame 8 {
              n1260 = local write "STROKE GAIN :"(w1579) -> ()
            }
            frame 9 {
            }
            frame 10 {
              n1261 = local write "Language Selection"(w1580) -> ()
            }
            frame 11 {
              n1262 = local write "CH-POWER +"(w1581) -> ()
            }
            frame 12 {
              n1263 = local write "CH-POWER -"(w1582) -> ()
            }
            frame 13 {
              n1264 = local write "CH-HEATER"(w1583) -> ()
            }
            frame 14 {
              n1265 = local write "CH-HUMIDITY WET"(w1584) -> ()
            }
            frame 15 {
              n1266 = local write "CH-HUMIDITY DRY"(w1585) -> ()
            }
            frame 16 {
            }
            frame 17 {
              n1267 = local write "AIR TEMP INTERCEPT:"(w1586) -> ()
            }
            frame 18 {
              n1268 = local write "TEMP INTERCEPT:"(w1587) -> ()
            }
            frame 19 {
              n1269 = local write "S.NO"(w1588) -> ()
            }
            frame 20 {
              n1270 = local write "Com Port 3"(w1589) -> ()
            }
            frame 21 {
            }
            frame 22 {
              n1271 = local write "C3 :"(w1590) -> ()
            }
            frame 23, Default {
            }
          }
        }
      }
    }
    n1272 = Select(t=u32 2500 ("milliseconds to wait"), s=w1544, f=u32 500 ("milliseconds to wait")) -> (s? t:f=w1542:u32)
    n1273 = Multiply(x=w1547, y=w1542) -> (x*y=w1549:dbl)
    n1274 = property on="Time slide" class="Slide (strict)"("Visible"=w1538) -> ()  [unwired: 2 in, 2 out]
    n1275 = call "Elapsed Time2"("Time Target (s)"=w1549, "Auto Reset"=TRUE) -> ("Time has Elapsed"=w1539:bool)  [unwired: 10 in, 7 out]
    n1276 = case shown="True" w1539 {
      frame False {
      }
      frame True {
        n1277 = stacked-sequence {
          frame #0 {
            # "DATA PROCESSING"
            # "115 mV/N"
            n1278 = local read "Sample Temperature"() -> (w1591:dbl)
            "TEMP 2" <- w1591
            "TEMP 3" <- w1591
            n1279 = local read "RH Numeric:"() -> (w1598:dbl)
            n1280 = local read "HUMIDITY:"() -> (w1599:dbl)
            n1281 = local read "FRICVALZ"() -> (w1610:dbl)
            n1282 = local read "Friction"() -> (w1594:dbl)
            n1283 = local write "TEMP"(w1591) -> ()
            n1284 = Multiply(x=w1598, y=w1599) -> (x*y=→"Humidity ( %RH )" →"Hum" →"Hum 2":dbl)
            n1285 = Subtract(x=w1594, y=w1610) -> (x-y=w1605:dbl)
            "FF 2" <- w1605
            "FF 4" <- w1605
            n1286 = local read "Ambient Temperature"() -> (→"AIR TEMP":dbl)
            n1287 = local read "TEMP"() -> (w1609:dbl)
            n1288 = local write "FF 3"(w1605) -> ()
            n1289 = Compound Arithmetic op=OR("FRICVALZ 4", "FRICVALZ 3", "FRICVALZ 2") -> (w1601:bool)
            n1290 = case shown="True" w1601 {
              tunnel: w1594 -> [_ w1616]
              frame False {
